vi "Construct Event State Change Callback.vi"(8 "error in (no error)":errorcluster) -> (0 "error out":errorcluster, 2 "Connection State Event Ref":refnum<user-event>, 3 "EventConnectionCallback out":refnum<class "EventConnectionCallback.lvclass">)   [LabVIEW 2020, in "EventConnectionCallback.lvclass"]
uses:
  <vilib>/gpm_packages/@cs/Network-interface/Examples/EventConnectionCallback/EventConnectionCallback.lvclass
  <vilib>/gpm_packages/@cs/Network-interface/Examples/EventConnectionCallback/ConnectionStateType.ctl
  <vilib>/gpm_packages/@cs/Network-interface/Examples/EventConnectionCallback/EventConnectionCallback.lvclass/EventConnectionCallback.ctl
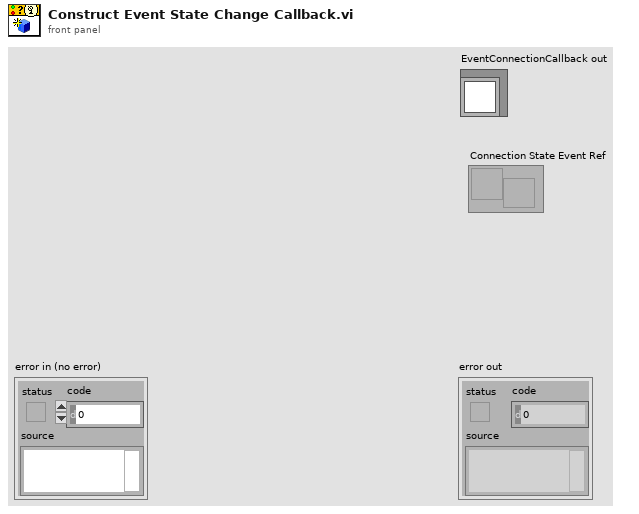
[diagram p1: front panel]
types:
  T1 = typedef "EventConnectionCallback.lvclass/ConnectionStateType.ctl" = cluster{"Connection ID":string, "State":bool}
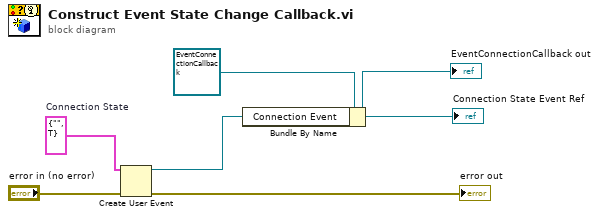
[diagram p0: block diagram]
diagram:
  w5 = T1 {"Connection ID"="", "State"=TRUE}  # Connection State
  n1 = Create User Event(user event datatype=w5, error in="error in (no error)") -> (user event=w1:refnum<user-event>, error out=→"error out":errorcluster)
  "Connection State Event Ref" <- w1
  n2 = Bundle By Name(cluster=refnum<class "EventConnectionCallback.lvclass"> refnum ("EventConnectionCallback in"), "Connection Event"=w1) -> (→"EventConnectionCallback out":refnum<class "EventConnectionCallback.lvclass">)
